vi "Create.vi"(8 "error in (no error)":errorcluster) -> (0 "error out":errorcluster, 3 "Parallell Test Runner out":refnum<class "Parallell Test Runner.lvclass">)   [LabVIEW 2020, in "Parallell Test Runner.lvclass"]
uses:
  Parallell Test Runner.lvclass
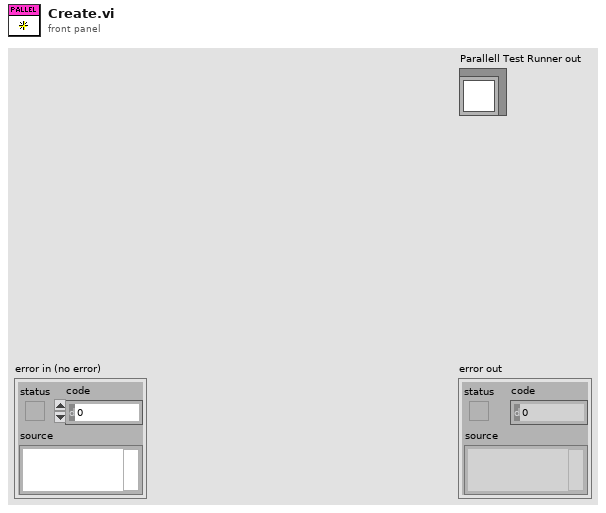
[diagram p1: front panel]
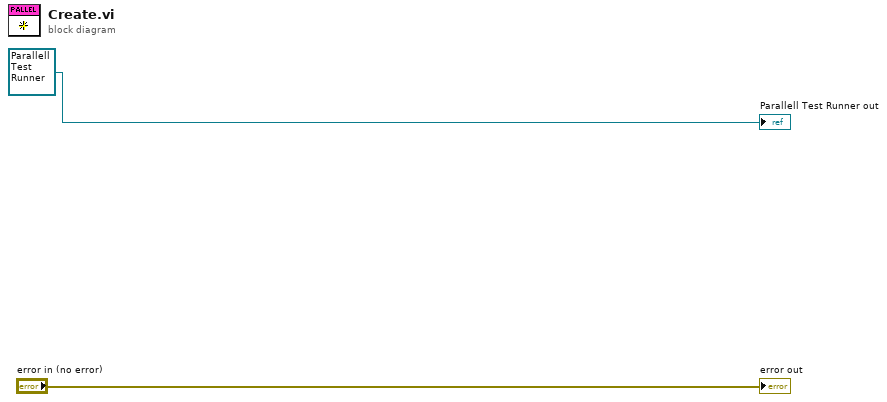
[diagram p0: block diagram]
diagram:
  "error out" <- "error in (no error)"
  "Parallell Test Runner out" <- refnum<class "Parallell Test Runner.lvclass"> refnum ("Parallell Test Runner in")
